vi "autosave_9234x2_9215trs.vi"() -> ()   [LabVIEW 2022 SP3]
uses:
  <vilib>/Utility/sysdir.llb/System Directory Type.ctl
  <vilib>/express/express analysis/Spectral/Block/exnSpectralBlock spectral measurements peak poly.vi
  <vilib>/express/express analysis/Spectral/Block/exnSpectralBlock spectral measurements peak DDT.vi
  <vilib>/express/express analysis/Spectral/XNode/ExpressSpectralMeasurementsBlockNode.xnode
panel:
  out "PEAK":dbl
  out "Trs 2":dynamicdata(graph)
  out "Use time (s)":dbl
  out "size(samples)":i32
  out "Filenames":string
  out "Trs":dynamicdata(graph)
  out "ON":bool
  out "DA":bool
  in  "enable save":bool=TRUE
  out "Queue":i32
  in  "Sample \nto Read":i32=6400
  in  "Sample\nRate":dbl=6400.0
  out "DW":bool
  in  "Show_FFT":bool=TRUE
  out "DAQ Stoped":bool
  in  "Stop":bool
  out "All":dynamicdata(graph)
  out "C1-0":dynamicdata(graph)
  out "C2-0":dynamicdata(graph)
  out "C1-1":dynamicdata(graph)
  out "C2-1":dynamicdata(graph)
  out "C1-2":dynamicdata(graph)
  out "C2-2":dynamicdata(graph)
  out "C1-3":dynamicdata(graph)
  out "C2-3":dynamicdata(graph)
  # "使用前請先確認 \nDAQ 擷取卡設定"
  # "本頁畫面顯示為 觸發後訊號"
  # "FFT Filter by useing High-pass with Lower Cut-Off (Hz)"
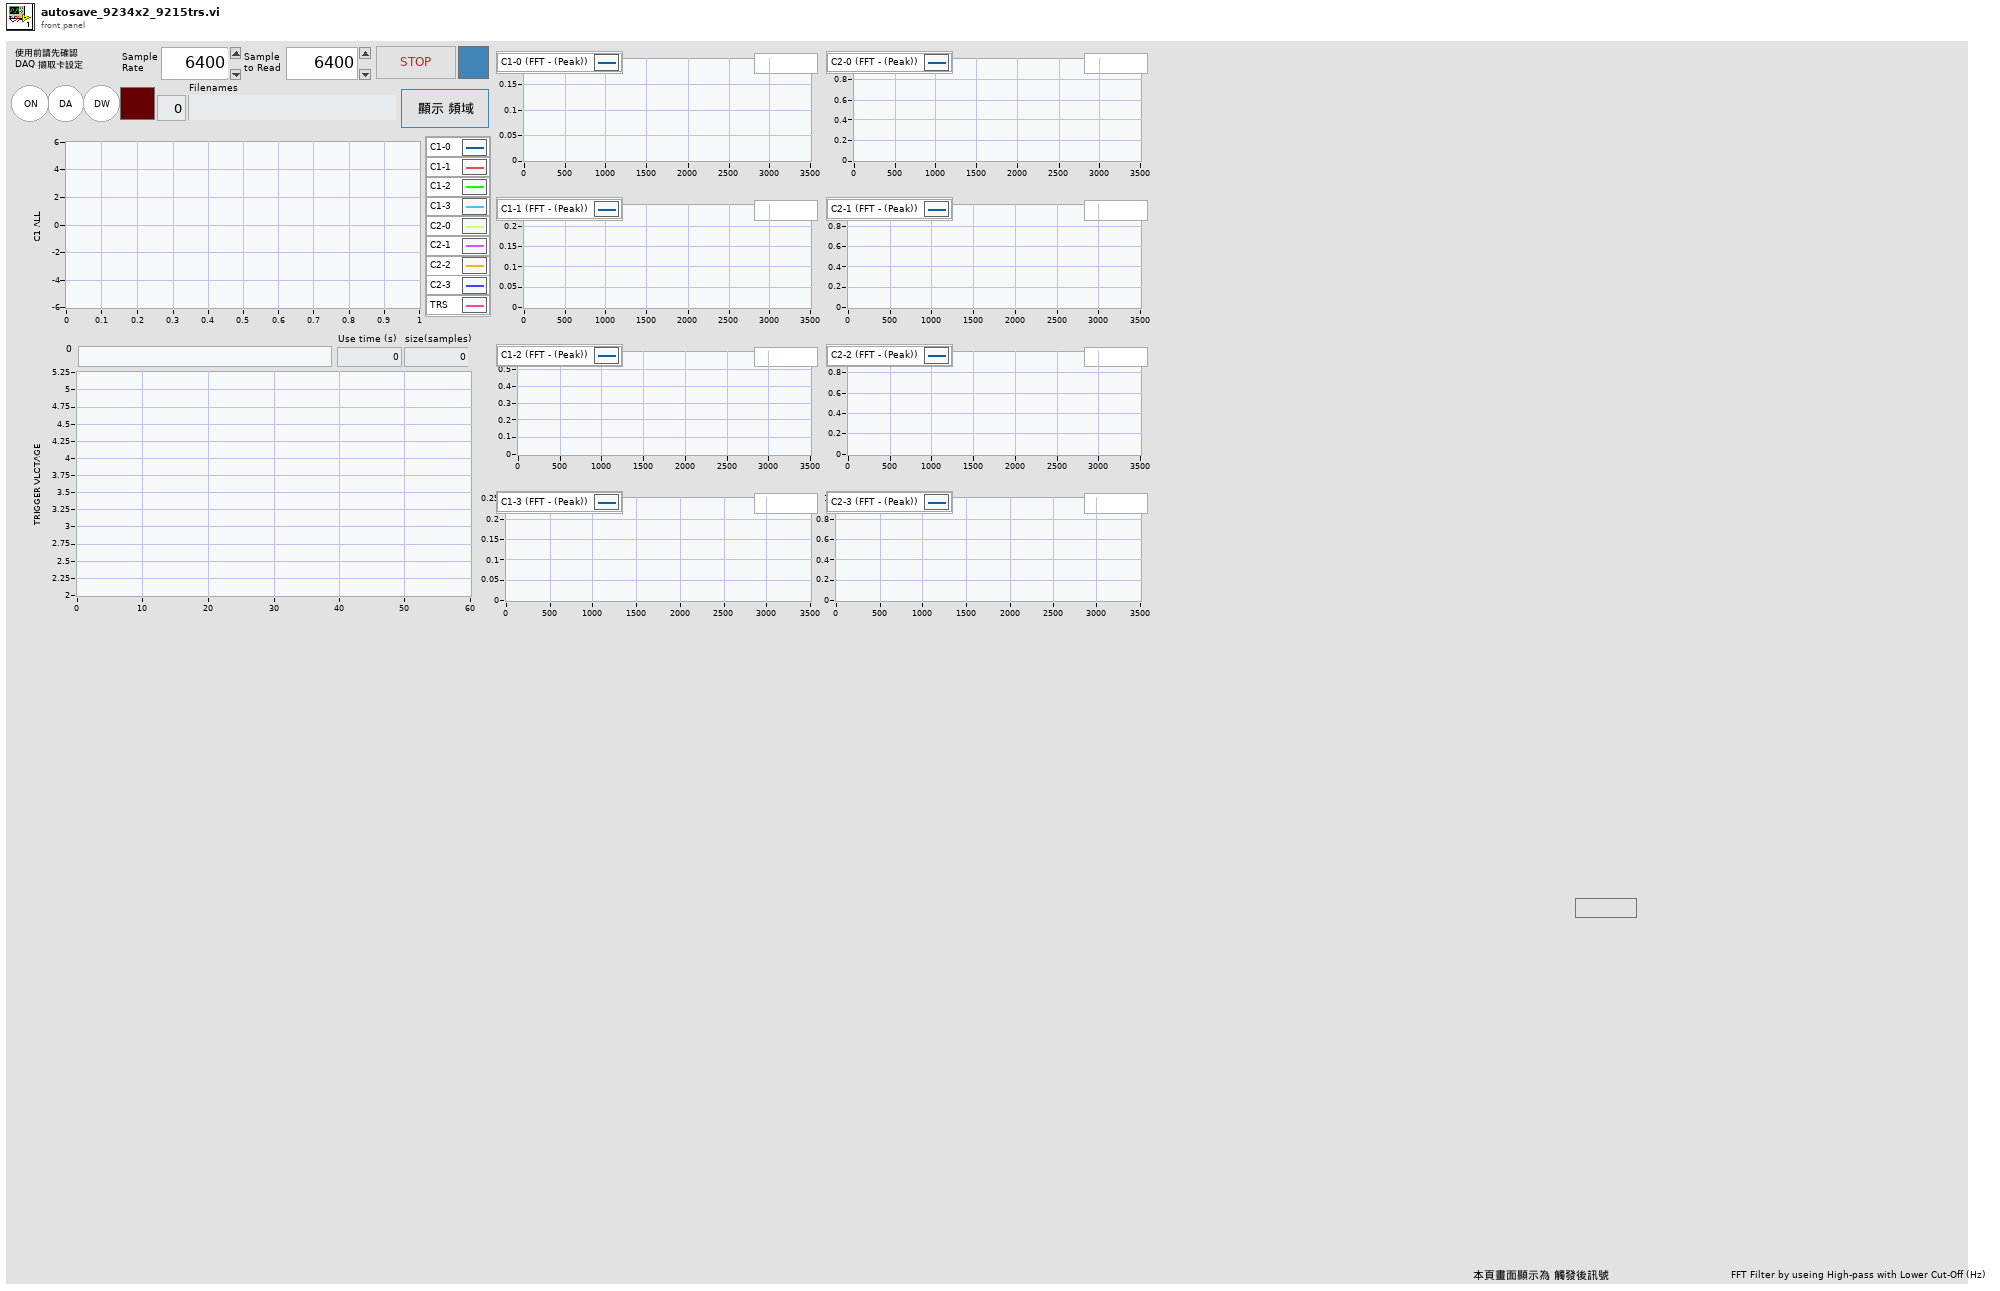
[diagram p1: front panel]
types:
  T1 = enum8{"Enabled", "Disabled", "Disabled and Grayed Out"}
  T2 = typedef "System Directory Type.ctl" = i32
  T3 = cluster{"task out":refnum<k21>, "data":dynamicdata}
  T4 = cluster{"averaging mode":u16, "weighting mode":u16, "number of averages":u32}
  T5 = cluster{"dB On (F)":bool, "unwrap phase (F)":bool, "convert to degree (F)":bool}
  T6 = enum16{"open", "open or create", "create or replace", "create", "open (read-only)"}
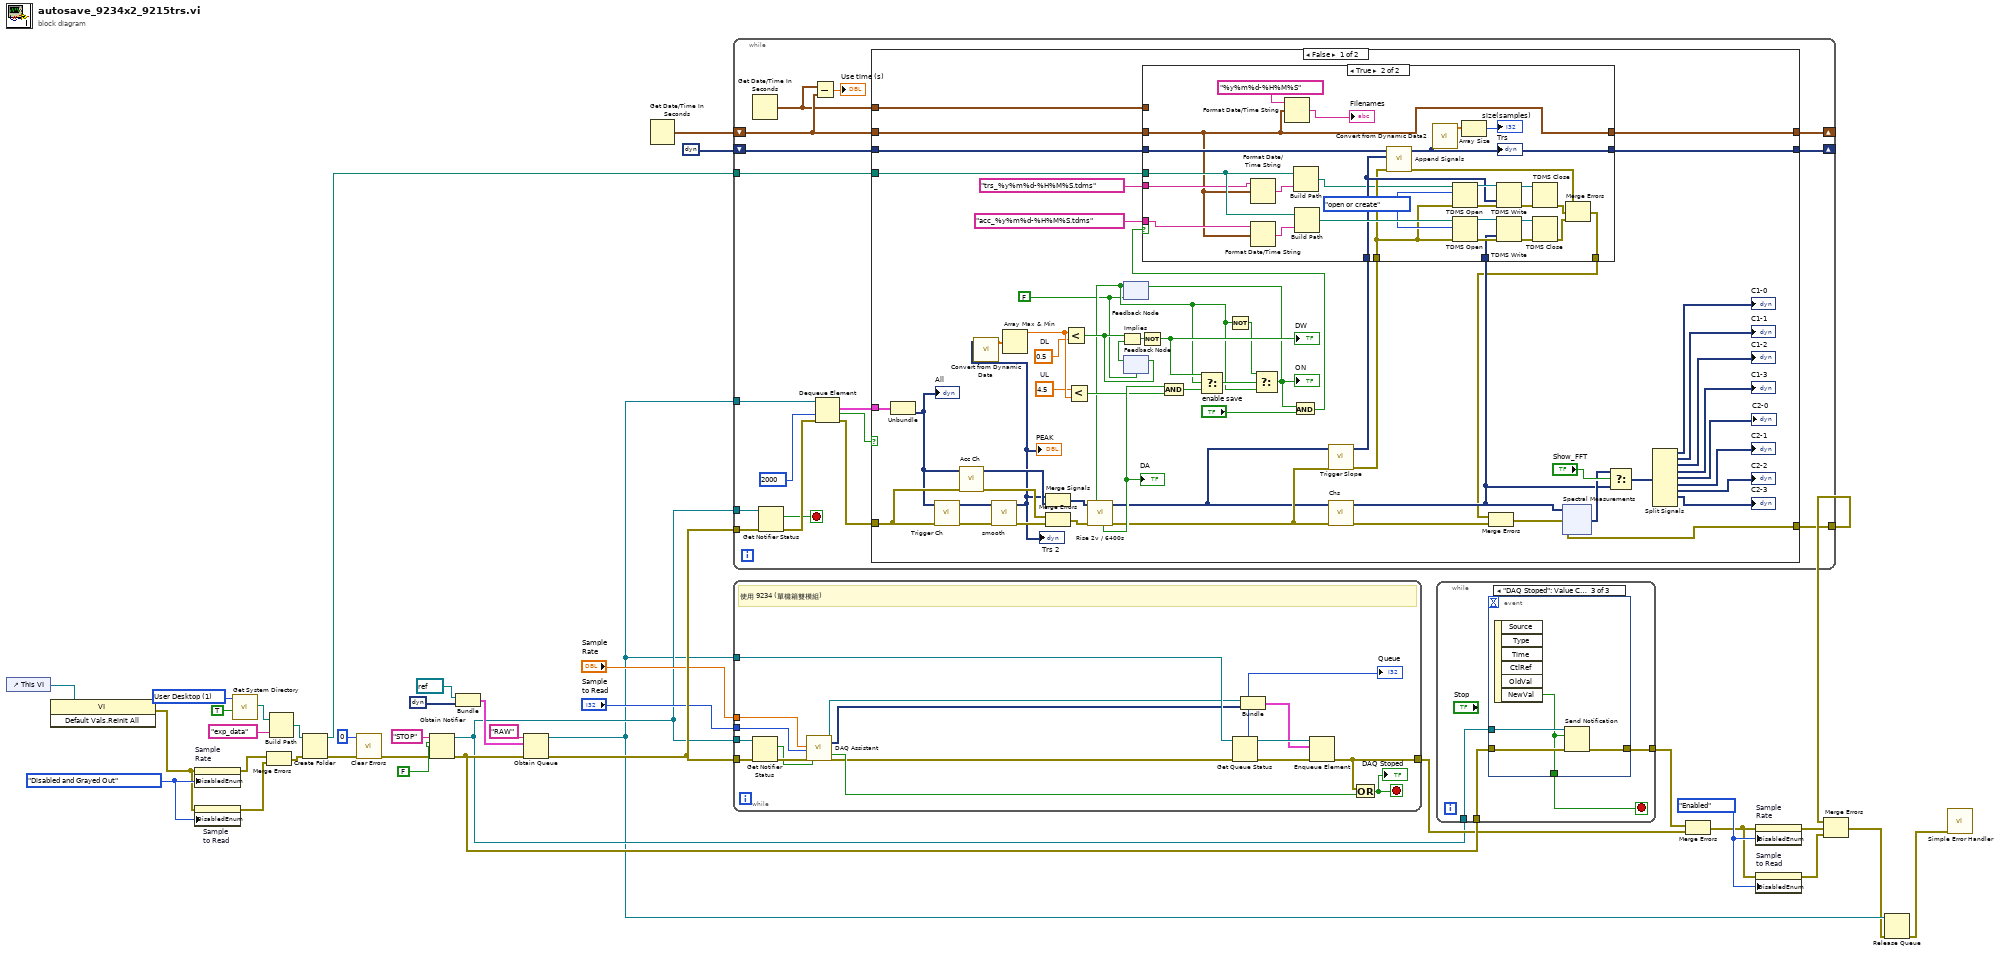
[diagram p0: block diagram]
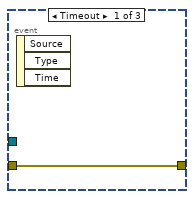
[diagram p2: hidden frame]
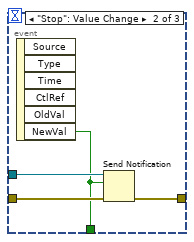
[diagram p3: hidden frame]
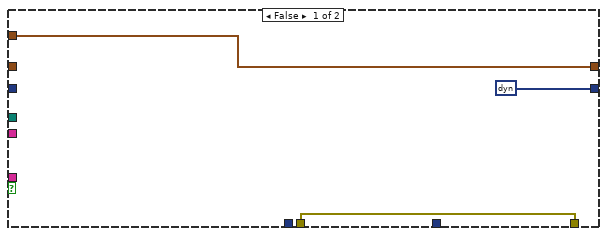
[diagram p4: hidden frame]
diagram:
  w12 = T1."Enabled" ("Disabled")
  w16 = T1."Disabled and Grayed Out" ("Disabled")
  w26 = T2 1 items=["User Home"=0, "User Desktop"=1, "User Documents"=2, "User Application Data"=3, "User Preferences"=4, "User Temporary"=5, "Public Documents"=6, "Public Application Data"=7, "Public Preferences"=8, "Public Cache"=13, "System Core Libraries"=9, "System Installed Libraries"=10, "Application Files"=11, "Boot Volume Root"=12] ("system directory type")
  n1 = control-ref of="This VI"() -> (w2:refnum<vi>)
  n2 = invoke class="VI" method="Default Vals.Reinit All"(reference=w2) -> (error out=w1:errorcluster)  [unwired: 2 in, 2 out]
  n3 = property on="Sample\nRate" class="DigNum (strict)"(error in=w1, "DisabledEnum"=w16) -> (error out=w15:errorcluster)  [unwired: 1 in, 1 out]
  n4 = property on="Sample \nto Read" class="DigNum (strict)"(error in=w1, "DisabledEnum"=w16) -> (error out=w13:errorcluster)  [unwired: 1 in, 1 out]
  n5 = call <vilib>:"Get System Directory.vi"("create directory if not found? (F)"=TRUE, "system directory type"=w26) -> ("system directory"=w28:path)  [unwired: 9 in]
  n6 = Merge Errors(w15, w13) -> (w14:errorcluster)
  n7 = Build Path(base path=w28, name or relative path="exp_data") -> (appended path=w22:path)
  n8 = Create Folder(path (use dialog)=w22, error in=w14) -> (created path=w21:path, error out=w24:errorcluster)  [unwired: 1 in, 1 out]
  n9 = call <vilib>:"Clear Errors.vi"("error in (no error)"=w24, "specific error code to clear (0: all)"=0) -> ("error out"=w23:errorcluster)  [unwired: 4 in, 1 out]
  n10 = Obtain Notifier(name (unnamed)="STOP", notification data type=FALSE, error in (no error)=w23) -> (notifier out=w17:refnum<notifier>, error out=w20:errorcluster)  [unwired: 1 in, 1 out]
  n11 = Bundle("task out"=refnum<k21> refnum, "data"=dynamicdata []) -> (w30:T3)  [unwired: 1 in]
  n12 = Obtain Queue(name (unnamed)="RAW", element data type=w30, error in (no error)=w20) -> (queue out=w8:refnum<queue>, error out=w38:errorcluster)  [unwired: 2 in, 1 out]
  n13 = Get Date/Time In Seconds() -> (seconds since 1Jan1904=w4:timestamp)
  n14 = while {
    tunnel: w38 -> [w55]
    tunnel: w17 -> [w53]
    tunnel: w8 -> [w52]
    shift-right: [w46] -> _
    shift-left: w4 -> [w47]
    tunnel: w21 -> [w45]
    tunnel: [w44] -> w6
    shift-right: [w41] -> _
    shift-left: dynamicdata [] ("Waveform Graph") -> [w42]
    stop <- w43 stop-if-true
    n15 = Get Date/Time In Seconds() -> (seconds since 1Jan1904=w40:timestamp)
    n16 = Get Notifier Status(notifier=w53, error in (no error)=w55) -> (current notification=w43:bool, error out=w54:errorcluster)  [unwired: 3 out]
    n17 = Subtract(x=w40, y=w47) -> (x-y=→"Use time (s)":dbl)
    n18 = Dequeue Element(queue=w52, timeout in ms (-1)=2000, error in (no error)=w54) -> (element=w49:T3, timed out?=w50:bool, error out=w48:errorcluster)  [unwired: 1 out]
    n19 = case shown="False" w50 {
      tunnel: w49 -> [w112 _]
      tunnel: w48 -> [w59 w158]
      tunnel: w47 -> [w105 w157]
      tunnel: [w69 w157] -> w46
      tunnel: w45 -> [w104 _]
      tunnel: [w111 w158] -> w44
      tunnel: w42 -> [w107 w156]
      tunnel: [w106 w156] -> w41
      tunnel: w40 -> [w70 _]
      frame False {
        w79 = FALSE
        w78 = 4.5  # UL
        w77 = 0.5  # DL
        n20 = Unbundle(w112) -> ("data"=w58:dynamicdata)  [unwired: 1 out]
        "All" <- w58
        n21 = call "Trigger Ch"("error in (no error)"=w59, "Signals"=w58) -> ("error out"=w63:errorcluster, "Signal Out"=w65:dynamicdata)  [unwired: 8 in]
        n22 = call "Acc Ch"("error in (no error)"=w59, "Signals"=w58) -> ("error out"=w61:errorcluster, "Signal Out"=w64:dynamicdata)  [unwired: 8 in]
        n23 = call "smooth"("error in (no error)"=w63, "Signal"=w65) -> ("error out"=w62:errorcluster, "Filtered Signal"=w57:dynamicdata)  [unwired: 8 in]
        "Trs 2" <- w57
        "PEAK" <- w57
        n24 = call "Convert from Dynamic Data"("Dynamic Data Type"=w57) -> ("Array"=w86:dbl[])  [unwired: 3 in]
        n25 = Array Max & Min(array=w86) -> (max value=w84:dbl)  [unwired: 3 out]
        n26 = Merge Signals(w57, w64) -> (w56:dynamicdata)
        n27 = Merge Errors(w61, w62) -> (w60:errorcluster)
        n28 = Less?(x=w84, y=w77) -> (x < y?=w87:bool)
        n29 = Less?(x=w78, y=w84) -> (x < y?=w83:bool)
        n30 = feedback #1(w79) -> (w82:bool)
        n31 = call "Rise 2v / 6400s"("Manual Trigger"=w82, "error in (no error)"=w60, "Signals"=w56) -> ("error out"=w76:errorcluster, "Triggered Signals"=w75:dynamicdata, "Data Available"=w91:bool)  [unwired: 5 in, 1 out]
        "DA" <- w91
        n32 = feedback #2(w79) -> (w88:bool)
        n33 = Implies(1:w88, 2:w87) -> (0:w89:bool)
        n34 = feedback-in #2(w87) -> ()
        n35 = Not(x=w89) -> (.not. x?=w92:bool)
        "DW" <- w92
        n36 = And(x=w91, y=w83) -> (x .and. y?=w81:bool)
        n37 = Select(t=w92, s=w82, f=w81) -> (s? t:f=w85:bool)
        n38 = Not(x=w82) -> (.not. x?=w80:bool)
        n39 = Select(t=w80, s=w85, f=w82) -> (s? t:f=w73:bool)
        "ON" <- w73
        n40 = feedback-in #1(w73) -> ()
        n41 = And(x=w73, y="enable save") -> (x .and. y?=w68:bool)
        n42 = call "Trigger Slope"("error in (no error)"=w76, "Signals"=w75) -> ("error out"=w72:errorcluster, "Signal Out"=w74:dynamicdata)  [unwired: 8 in]
        n43 = call "Chs"("error in (no error)"=w76, "Signals"=w75) -> ("error out"=w108:errorcluster, "Signal Out"=w93:dynamicdata)  [unwired: 8 in]
        n44 = case shown="True" w68 {
          tunnel: w107 -> [_ w145]
          tunnel: [dynamicdata [] ("Waveform Graph") w144] -> w106
          tunnel: w105 -> [_ w118]
          tunnel: w104 -> [_ w143]
          tunnel: w93 -> [_ w134]
          tunnel: w74 -> [_ w126]
          tunnel: w72 -> [w115 w125]
          tunnel: [w115 w122] -> w71
          tunnel: w70 -> [w114 _]
          tunnel: [w114 w118] -> w69
          tunnel: "acc_%y%m%d-%H%M%S.tdms" ("string") -> [_ w121]
          tunnel: "trs_%y%m%d-%H%M%S.tdms" ("string") -> [_ w120]
          frame False {
          }
          frame True {
            w127 = T6."open or create" ("operation (0:open)")
            n45 = Format Date/Time String(time format string (%c)=w120, seconds (now)=w118) -> (date/time string=w116:string)  [unwired: 1 in]
            n46 = Format Date/Time String(time format string (%c)=w121, seconds (now)=w118) -> (date/time string=w117:string)  [unwired: 1 in]
            n47 = Format Date/Time String(time format string (%c)="%y%m%d-%H%M%S", seconds (now)=w118) -> (date/time string=→"Filenames":string)  [unwired: 1 in]
            n48 = Build Path(base path=w143, name or relative path=w116) -> (appended path=w124:path)
            n49 = Build Path(base path=w143, name or relative path=w117) -> (appended path=w135:path)
            n50 = call "Append Signals"("error in (no error)"=w125, "Input Signal B"=w126, "Input Signal A"=w145) -> ("error out"=w123:errorcluster, "Appended Signals"=w144:dynamicdata)  [unwired: 7 in]
            "Trs" <- w144
            n51 = call "Convert from Dynamic Data2"("Dynamic Data Type"=w144) -> ("Array"=w141:dbl[])  [unwired: 3 in]
            n52 = TDMS Open(8:w125, 10:w127, 11:w124) -> (0:w131:errorcluster, 3:w130:refnum<k34>)  [unwired: 4 in]
            n53 = TDMS Open(8:w125, 10:w127, 11:w135) -> (0:w138:errorcluster, 3:w139:refnum<k34>)  [unwired: 4 in]
            n54 = Array Size(array=w141) -> (size(s)=→"size(samples)":i32)
            n55 = TDMS Write(0:w130, 9:w126, 11:w131) -> (4:w132:refnum<k34>, 15:w133:errorcluster)  [unwired: 3 in, 2 out]
            n56 = TDMS Write(0:w139, 9:w134, 11:w138) -> (4:w137:refnum<k34>, 15:w136:errorcluster)  [unwired: 3 in, 2 out]
            n57 = TDMS Close(8:w133, 11:w132) -> (0:w129:errorcluster)  [unwired: 1 out]
            n58 = TDMS Close(8:w136, 11:w137) -> (0:w128:errorcluster)  [unwired: 1 out]
            n59 = Merge Errors(w123, w129, w128) -> (w122:errorcluster)
          }
        }
        n60 = Merge Errors(w71, w108) -> (w94:errorcluster)
        n61 = xnode ("Spectral Measurements")("Signals"=w93, "error in (no error)"=w94) -> ("FFT - (Peak)"=w109:dynamicdata, "error out"=w111:errorcluster)  [unwired: 1 out]
        n62 = Select(t=w109, s="Show_FFT", f=w93) -> (s? t:f=w103:dynamicdata)
        n63 = Split Signals(w103) -> (→"C1-0":dynamicdata, →"C1-1":dynamicdata, →"C1-2":dynamicdata, →"C1-3":dynamicdata, →"C2-0":dynamicdata, →"C2-1":dynamicdata, →"C2-2":dynamicdata, →"C2-3":dynamicdata)  [unwired: 9 in, 1 out]
      }
      frame True {
      }
    }
  }
  n64 = while {
    tunnel: [w171] -> w18
    tunnel: w8 -> [w168]
    tunnel: w38 -> [w167]
    tunnel: w17 -> [w166]
    tunnel: "Sample \nto Read" -> [w162]
    tunnel: "Sample\nRate" -> [w161]
    stop <- w169 stop-if-true
    # "使用 9234 (單機箱雙模組)"
    n65 = Get Notifier Status(notifier=w166, error in (no error)=w167) -> (current notification=w174:bool, error out=w175:errorcluster)  [unwired: 3 out]
    n66 = call "DAQ Assistant"("rate"=w161, "number of samples"=w162, "error in"=w175, "stop (F)"=w174) -> ("task out"=w164:refnum<k21>, "data"=w160:dynamicdata, "stopped"=w173:bool, "error out"=w159:errorcluster)  [unwired: 12 in]
    n67 = Get Queue Status(queue=w168, error in (no error)=w159) -> (queue out=w165:refnum<queue>, error out=w172:errorcluster, # elements in queue=→"Queue":i32)  [unwired: 1 in, 5 out]
    n68 = Bundle("task out"=w164, "data"=w160) -> (w163:T3)  [unwired: 1 in]
    n69 = Enqueue Element(queue=w165, element=w163, error in (no error)=w172) -> (error out=w171:errorcluster)  [unwired: 1 in, 2 out]
    n70 = Compound Arithmetic op=OR(w171, w173) -> (w169:bool)
    "DAQ Stoped" <- w169
  }
  n71 = while {
    tunnel: w20 -> [w179]
    tunnel: [w178] -> w19
    tunnel: w17 -> [w177]
    stop <- w176 stop-if-true
    n72 = event shown="[2] \"DAQ Stoped\": Value Change" {
      selector: _ -> [_ _ _]
      dyn-events: _ -> [_ _ _]
      timeout: _ -> [_ _ _]
      tunnel: w179 -> [w180 w184 w188]
      tunnel: [w180 w183 w187] -> w178
      tunnel: w177 -> [_ w182 w186]
      tunnel: [_ w181 w185] -> w176
      event Timeout {
        n73 = event-data() -> ()  [unwired: 1 in, 3 out]
      }
      event "Stop": Value Change {
        n74 = event-data() -> ("NewVal"=w181:bool)  [unwired: 1 in, 5 out]
        n75 = Send Notification(notification=w181, notifier=w182, error in (no error)=w184) -> (error out=w183:errorcluster)  [unwired: 1 out]
      }
      event "DAQ Stoped": Value Change {
        n76 = event-data() -> ("NewVal"=w185:bool)  [unwired: 1 in, 5 out]
        n77 = Send Notification(notification=w185, notifier=w186, error in (no error)=w188) -> (error out=w187:errorcluster)  [unwired: 1 out]
      }
    }
  }
  n78 = Merge Errors(w19, w18) -> (w9:errorcluster)
  n79 = property on="Sample\nRate" class="DigNum (strict)"(error in=w9, "DisabledEnum"=w12) -> (error out=w11:errorcluster)  [unwired: 1 in, 1 out]
  n80 = property on="Sample \nto Read" class="DigNum (strict)"(error in=w9, "DisabledEnum"=w12) -> (error out=w10:errorcluster)  [unwired: 1 in, 1 out]
  n81 = Merge Errors(w6, w11, w10) -> (w5:errorcluster)
  n82 = Release Queue(queue=w8, error in (no error)=w5) -> (error out=w7:errorcluster)  [unwired: 1 in, 2 out]
  n83 = call <vilib>:"Simple Error Handler.vi"("error in (no error)"=w7) -> ()  [unwired: 4 in, 5 out]
